vi "Teleop - Robot Angle (SubVI).vi"(11 "yaw in":dbl) -> (2 "angle":dbl)   [LabVIEW 2019]
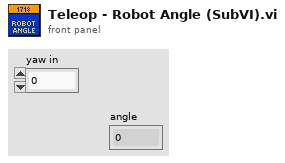
[diagram p1: front panel]
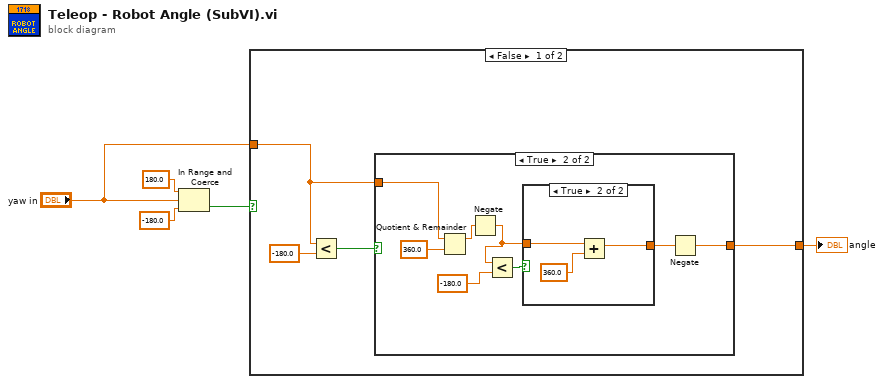
[diagram p0: block diagram]
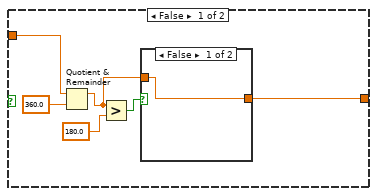
[diagram p2: hidden frame]
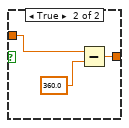
[diagram p3: hidden frame]
diagram:
  n1 = In Range and Coerce(upper limit=180.0, x="yaw in", lower limit=-180.0) -> (In Range?=w3:bool)  [unwired: 1 out]
  n2 = case shown="False" w3 {
    tunnel: [w6 w32] -> w4
    tunnel: "yaw in" -> [w7 w32]
    frame False {
      n3 = Less?(x=w7, y=-180.0) -> (x < y?=w8:bool)
      n4 = case shown="True" w8 {
        tunnel: w7 -> [w14 w26]
        tunnel: [w13 w20] -> w6
        frame False {
          n5 = Quotient & Remainder(x=w14, y=360.0) -> (x-y*floor(x/y)=w10:dbl)  [unwired: 1 out]
          n6 = Greater?(x=w10, y=180.0) -> (0:w11:bool)
          n7 = case shown="False" w11 {
            tunnel: [w16 w18] -> w13
            tunnel: w10 -> [w16 w17]
            frame False {
            }
            frame True {
              n8 = Subtract(x=w17, y=360.0) -> (x-y=w18:dbl)
            }
          }
        }
        frame True {
          n9 = Quotient & Remainder(x=w26, y=360.0) -> (x-y*floor(x/y)=w22:dbl)  [unwired: 1 out]
          n10 = Negate(x=w22) -> (-x=w23:dbl)
          n11 = Less?(x=w23, y=-180.0) -> (x < y?=w24:bool)
          n12 = case shown="True" w24 {
            tunnel: [w28 w30] -> w21
            tunnel: w23 -> [w28 w29]
            frame False {
            }
            frame True {
              n13 = Add(x=w29, y=360.0) -> (x+y=w30:dbl)
            }
          }
          n14 = Negate(x=w21) -> (-x=w20:dbl)
        }
      }
    }
    frame True {
    }
  }
  "angle" <- w4
